vi "Diplay Documentation Image.vi"(8 "error in (no error)":errorcluster, 11 "Image Name":string) -> (0 "error out":errorcluster)   [LabVIEW 2019, in "Configuration Tool.lvlib"]
uses:
  Configuration Tool.lvlib
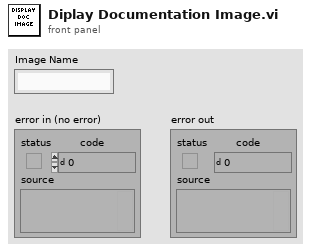
[diagram p1: front panel]
types:
  T1 = typedef "imagedata.ctl" = cluster{"image type":i32, "image depth":i32, "image":u8[], "mask":u8[], "colors":u32[], "Rectangle":cluster{"left":i16, "top":i16, "right":i16, "bottom":i16}}
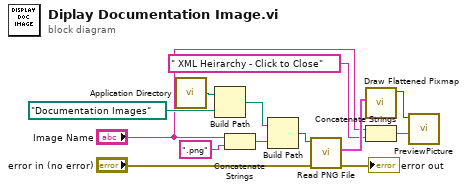
[diagram p0: block diagram]
diagram:
  n1 = call <vilib>:"Application Directory.vi"() -> ("Application Directory"=w13:path)
  n2 = Build Path(base path=w13, name or relative path=path "Documentation Images" ("Path")) -> (appended path=w9:path)
  n3 = Concatenate Strings("Image Name", ".png" ("string")) -> (w1:string)
  n4 = Build Path(base path=w9, name or relative path=w1) -> (appended path=w8:path)
  n5 = call <vilib>:"Read PNG File.vi"("error in (no error)"="error in (no error)", "path to PNG file"=w8) -> ("error out"=→"error out":errorcluster, "image data"=w12:T1)  [unwired: 7 in, 1 out]
  n6 = call <vilib>:"Draw Flattened Pixmap.vi"("image data"=w12) -> ("new picture"=w11:picture)  [unwired: 8 in]
  n7 = Concatenate Strings("Image Name", " XML Heirarchy - Click to Close" ("string")) -> (w4:string)
  n8 = call "PreviewPicture.vi"("Title"=w4, "2D Picture"=w11) -> ()  [unwired: 10 in]
